vi "Save Refs to INI.vi"(10 "Configuration file path":path, 11 "Array of Control References":refnum<vi>[](array[refnum])) -> ()   [LabVIEW 2019]
uses:
  <vilib>/Utility/config.llb/Write Key (Path).vi
  <vilib>/Utility/config.llb/Write Key (Boolean).vi
  <vilib>/Utility/config.llb/Write Key (Double).vi
  <vilib>/Utility/config.llb/Write Key (String).vi
  <vilib>/Utility/config.llb/Write Key (I32).vi
  <vilib>/Utility/config.llb/Write Key (U32).vi
  <vilib>/Utility/config.llb/NI_LVConfig.lvlib
panel:
  out "Array out":string[](array[string])
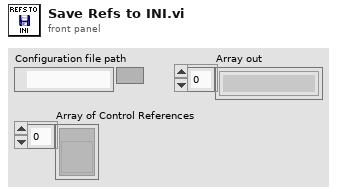
[diagram p1: front panel]
types:
  T1 = typedef "NI_LVConfig.lvlib/Config Data RefNum.ctl" = refnum<k1>
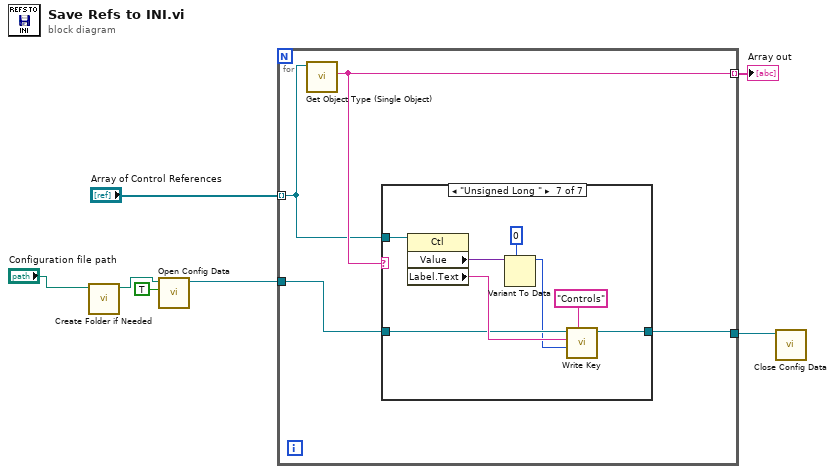
[diagram p0: block diagram]
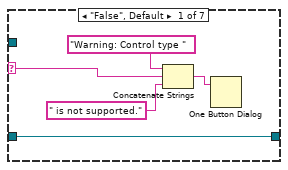
[diagram p2: hidden frame]
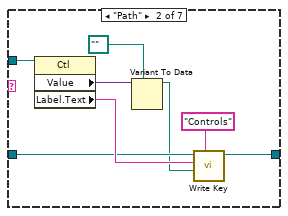
[diagram p3: hidden frame]
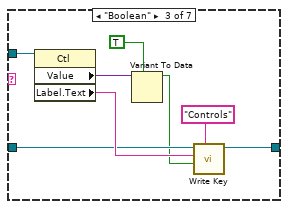
[diagram p4: hidden frame]
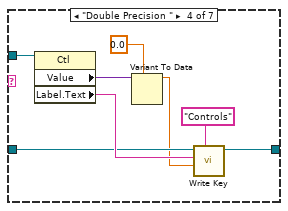
[diagram p5: hidden frame]
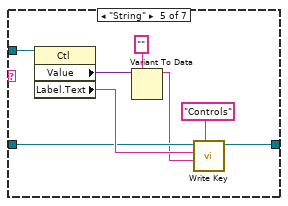
[diagram p6: hidden frame]
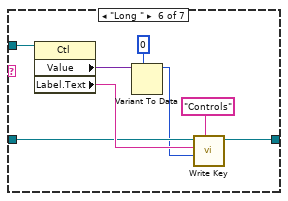
[diagram p7: hidden frame]
diagram:
  n1 = call "Create Folder if Needed.vi"("Settings File Path"="Configuration file path") -> ("File Path Out"=w1:path)  [unwired: 10 in]
  n2 = call <vilib>:"Open Config Data.vi"("create file if necessary (T)"=TRUE, "configuration file path"=w1) -> ("refnum"=w7:T1)  [unwired: 7 in, 2 out]
  n3 = for {
    tunnel: "Array of Control References" -> [w8] mode=indexing
    tunnel: [w9] -> w4 mode=indexing
    tunnel: [w10] -> w6
    tunnel: w7 -> [w11]
    n4 = call "Get Object Type (Single Object).vi"("Object Reference"=w8) -> ("Object Type"=w9:string)  [unwired: 8 in, 2 out]
    n5 = case shown="\"Unsigned Long \"" w9 {
      selector: w9 -> [w14 _ _ _ _ _ _]
      tunnel: w11 -> [w16 w21 w29 w37 w45 w53 w61]
      tunnel: [w16 w20 w28 w36 w44 w52 w60] -> w10
      tunnel: w8 -> [_ w17 w25 w33 w42 w50 w58]
      frame "False", Default {
        n6 = Concatenate Strings("Warning: Control type " ("string"), w14, " is not supported." ("string")) -> (w12:string)
        n7 = One Button Dialog(message=w12) -> ()  [unwired: 1 in, 1 out]
      }
      frame "Path" {
        n8 = property class="Ctl"(reference=w17) -> ("Value"=w24:variant, "Label.Text"=w23:string)  [unwired: 1 in, 2 out]
        n9 = Variant To Data(type=path "", Variant=w24) -> (data=w18:path)  [unwired: 1 in, 1 out]
        n10 = call-poly <vilib>:"Write Key.vi"("section"="Controls", "value"=w18, "key"=w23, "refnum"=w21) -> ("refnum out"=w20:T1)  [unwired: 5 in, 2 out]
      }
      frame "Boolean" {
        n11 = property class="Ctl"(reference=w25) -> ("Value"=w32:variant, "Label.Text"=w31:string)  [unwired: 1 in, 2 out]
        n12 = Variant To Data(type=TRUE, Variant=w32) -> (data=w27:bool)  [unwired: 1 in, 1 out]
        n13 = call-poly <vilib>:"Write Key.vi"("section"="Controls", "value"=w27, "key"=w31, "refnum"=w29) -> ("refnum out"=w28:T1)  [unwired: 5 in, 2 out]
      }
      frame "Double Precision " {
        n14 = property class="Ctl"(reference=w33) -> ("Value"=w40:variant, "Label.Text"=w39:string)  [unwired: 1 in, 2 out]
        n15 = Variant To Data(type=0.0, Variant=w40) -> (data=w35:dbl)  [unwired: 1 in, 1 out]
        n16 = call-poly <vilib>:"Write Key.vi"("section"="Controls", "value"=w35, "key"=w39, "refnum"=w37) -> ("refnum out"=w36:T1)  [unwired: 5 in, 2 out]
      }
      frame "String" {
        n17 = property class="Ctl"(reference=w42) -> ("Value"=w48:variant, "Label.Text"=w47:string)  [unwired: 1 in, 2 out]
        n18 = Variant To Data(type="", Variant=w48) -> (data=w43:string)  [unwired: 1 in, 1 out]
        n19 = call-poly <vilib>:"Write Key.vi"("section"="Controls", "value"=w43, "key"=w47, "refnum"=w45) -> ("refnum out"=w44:T1)  [unwired: 5 in, 2 out]
      }
      frame "Long " {
        n20 = property class="Ctl"(reference=w50) -> ("Value"=w56:variant, "Label.Text"=w55:string)  [unwired: 1 in, 2 out]
        n21 = Variant To Data(type=0 ("Integer - Long"), Variant=w56) -> (data=w51:i32)  [unwired: 1 in, 1 out]
        n22 = call-poly <vilib>:"Write Key.vi"("section"="Controls", "value"=w51, "key"=w55, "refnum"=w53) -> ("refnum out"=w52:T1)  [unwired: 5 in, 2 out]
      }
      frame "Unsigned Long " {
        n23 = property class="Ctl"(reference=w58) -> ("Value"=w64:variant, "Label.Text"=w63:string)  [unwired: 1 in, 2 out]
        n24 = Variant To Data(type=u32 0 ("Integer - Unsigned Long"), Variant=w64) -> (data=w59:u32)  [unwired: 1 in, 1 out]
        n25 = call-poly <vilib>:"Write Key.vi"("section"="Controls", "value"=w59, "key"=w63, "refnum"=w61) -> ("refnum out"=w60:T1)  [unwired: 5 in, 2 out]
      }
    }
  }
  "Array out" <- w4
  n26 = call <vilib>:"Close Config Data.vi"("refnum"=w6) -> ()  [unwired: 9 in, 2 out]
